vi "Multiply.vi"(2 "SampleFreq":dbl, 7 "Array in":cdb[](array[numeric]), 13 "MultiplyFreq":dbl) -> (8 "Array out":cdb[](array[numeric]))   [LabVIEW 2020]
uses:
  <vilib>/Analysis/NI_AAL_Angle.lvlib
  <vilib>/Analysis/coordinate.llb/Wrap Angle (scalar).vi
  <vilib>/Analysis/NI_AALPro.lvlib
  <vilib>/Analysis/2dsp.llb/Inverse Complex FFT.vi
  <vilib>/Analysis/2dsp.llb/Complex FFT.vi
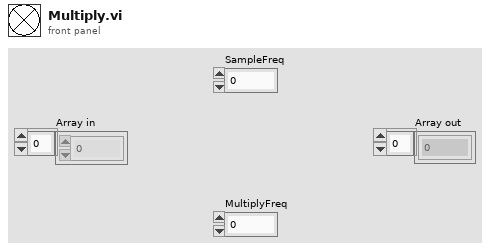
[diagram p1: front panel]
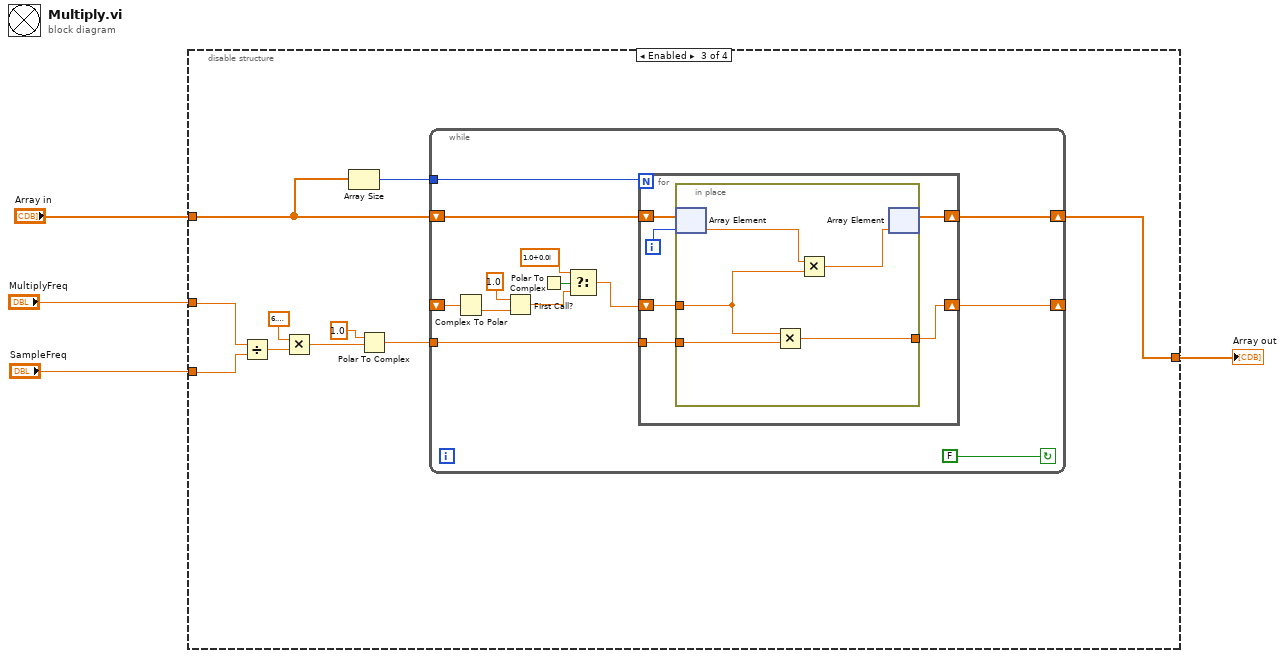
[diagram p0: block diagram]
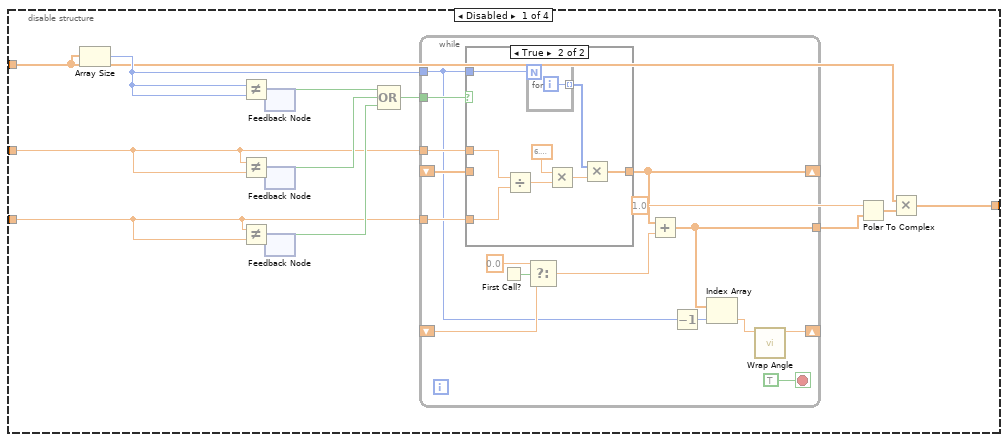
[diagram p2: hidden frame]
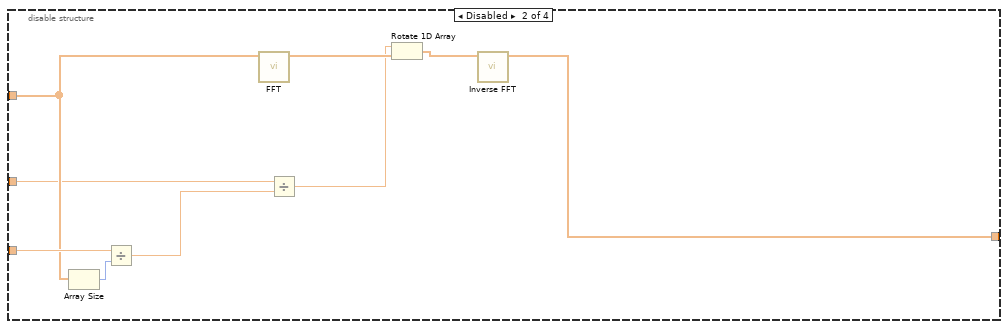
[diagram p4: hidden frame]
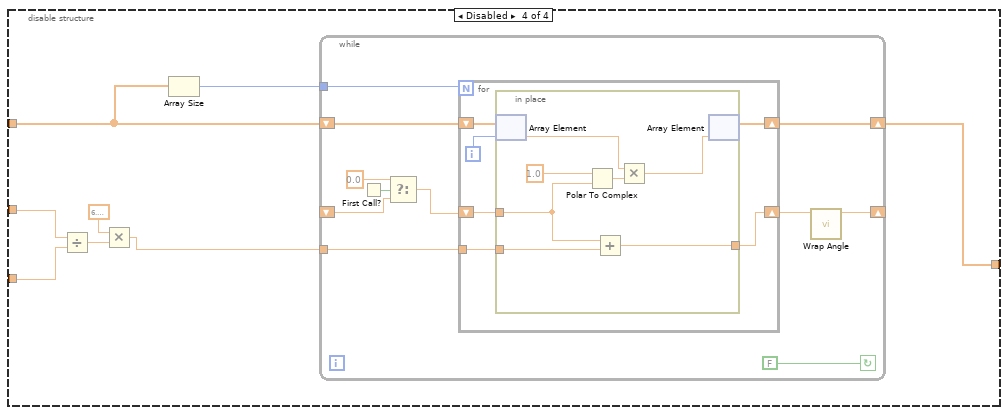
[diagram p5: hidden frame]
diagram:
  n1 = disable-structure shown="Enabled" {
    disable-tunnel: "MultiplyFreq" -> [w11 w50 w57 w89]
    disable-tunnel: "SampleFreq" -> [w10 w53 w58 w90]
    disable-tunnel: "Array in" -> [w6 w51 w62 w94]
    disable-tunnel: [w5 w45 w61 w93] -> w2
    frame Disabled {
      n2 = Array Size(array=w6) -> (size(s)=w12:i32)
      n3 = feedback #1() -> (w17:i32)  [unwired: 1 in]
      n4 = Not Equal?(x=w12, y=w17) -> (x != y?=w15:bool)
      n5 = feedback-in #1(w12) -> ()
      n6 = feedback #2() -> (w18:dbl)  [unwired: 1 in]
      n7 = Not Equal?(x=w11, y=w18) -> (x != y?=w14:bool)
      n8 = feedback-in #2(w11) -> ()
      n9 = feedback #3() -> (w19:dbl)  [unwired: 1 in]
      n10 = Not Equal?(x=w10, y=w19) -> (x != y?=w16:bool)
      n11 = feedback-in #3(w10) -> ()
      n12 = Compound Arithmetic op=OR(w15, w14, w16) -> (w13:bool)
      n13 = while {
        tunnel: w13 -> [w31]
        tunnel: w12 -> [w21]
        tunnel: w11 -> [w32]
        tunnel: w10 -> [w33]
        shift-right: [w26] -> _
        shift-left: _ -> [w30]
        shift-right: [w25] -> _
        shift-left: _ -> [w27]
        tunnel: [w20] -> w9
        stop <- TRUE stop-if-true
        n14 = case shown="True" w31 {
          tunnel: w21 -> [_ w43]
          tunnel: w33 -> [_ w40]
          tunnel: w32 -> [_ w39]
          tunnel: [w35 w36] -> w26
          tunnel: w30 -> [w35 _]
          frame False {
          }
          frame True {
            n15 = Divide(x=w39, y=w40) -> (x/y=w42:dbl)
            n16 = for {
              N: w43 -> [_]
              tunnel: [w44] -> w37 mode=indexing
              i -> [w44]
            }
            n17 = Multiply(x=6.283185307179586, y=w42) -> (x*y=w38:dbl)
            n18 = Multiply(x=w37, y=w38) -> (x*y=w36:dbl[])
          }
        }
        n19 = First Call?() -> (First Call?: T/F=w29:bool)
        n20 = Select(t=0.0, s=w29, f=w27) -> (s? t:f=w24:dbl)
        n21 = Add(x=w26, y=w24) -> (x+y=w20:dbl[])
        n22 = Decrement(x=w21) -> (x-1=w22:i32)
        n23 = Index Array(array=w20, index=w22) -> (element=w23:dbl)
        n24 = call-poly <vilib>:"Wrap Angle.vi"("angle in"=w23) -> ("angle out"=w25:dbl)  [unwired: 9 in, 1 out]
      }
      n25 = Polar To Complex(1:w9, 2:1.0 ("r")) -> (0:w7:cdb[])
      n26 = Multiply(x=w6, y=w7) -> (x*y=w5:cdb[])
    }
    frame Disabled {
      n27 = Array Size(array=w51) -> (size(s)=w52:i32)
      n28 = Divide(x=w53, y=w52) -> (x/y=w49:dbl)
      n29 = call-poly <vilib>:"FFT.vi"("X"=w51) -> ("FFT {X}"=w48:cdb[])  [unwired: 9 in, 1 out]
      n30 = Divide(x=w50, y=w49) -> (x/y=w46:dbl)
      n31 = Rotate 1D Array(1:w48, 2:w46) -> (0:w47:cdb[])
      n32 = call-poly <vilib>:"Inverse FFT.vi"("FFT {X}"=w47) -> ("X"=w45:cdb[])  [unwired: 9 in, 1 out]
    }
    frame Enabled {
      n33 = Divide(x=w57, y=w58) -> (x/y=w60:dbl)
      n34 = Multiply(x=6.283185307179586, y=w60) -> (x*y=w55:dbl)
      n35 = Array Size(array=w62) -> (size(s)=w63:i32)
      n36 = Polar To Complex(1:w55, 2:1.0 ("r")) -> (0:w54:cdb)
      n37 = while {
        tunnel: w63 -> [w75]
        tunnel: w54 -> [w73]
        shift-right: [w76] -> w61
        shift-left: w62 -> [w74]
        shift-right: [w68] -> _
        shift-left: _ -> [w67]
        stop <- FALSE continue-if-true
        n38 = Complex To Polar(r * e^(i*theta)=w67) -> (theta=w66:dbl)  [unwired: 1 out]
        n39 = Polar To Complex(1:w66, 2:1.0 ("r")) -> (0:w64:cdb)
        n40 = First Call?() -> (First Call?: T/F=w72:bool)
        n41 = Select(t=cdb 1.0+0.0i, s=w72, f=w64) -> (s? t:f=w69:cdb)
        n42 = for {
          N: w75 -> [_]
          shift-right: [w77] -> w76
          shift-left: w74 -> [w82]
          tunnel: w73 -> [w80]
          shift-right: [w79] -> w68
          shift-left: w69 -> [w78]
          i -> [w81]
          n43 = in-place {
            in-place-border: w80 -> [w87]
            in-place-border: [w84] -> w79
            in-place-border: w78 -> [w83]
            n44 = in-place-array #4(w82, w81) -> (w86:cdb)
            n45 = Multiply(x=w83, y=w87) -> (x*y=w84:cdb)
            n46 = Multiply(x=w86, y=w83) -> (x*y=w85:cdb)
            n47 = in-place-array #4(w85) -> (w77:cdb[])  [unwired: 1 out]
          }
        }
      }
    }
    frame Disabled {
      n48 = Divide(x=w89, y=w90) -> (x/y=w92:dbl)
      n49 = Multiply(x=6.283185307179586, y=w92) -> (x*y=w88:dbl)
      n50 = Array Size(array=w94) -> (size(s)=w95:i32)
      n51 = while {
        tunnel: w95 -> [w105]
        tunnel: w88 -> [w103]
        shift-right: [w106] -> w93
        shift-left: w94 -> [w104]
        shift-right: [w96] -> _
        shift-left: _ -> [w101]
        stop <- FALSE continue-if-true
        n52 = First Call?() -> (First Call?: T/F=w102:bool)
        n53 = Select(t=0.0, s=w102, f=w101) -> (s? t:f=w98:dbl)
        n54 = for {
          N: w105 -> [_]
          shift-right: [w107] -> w106
          shift-left: w104 -> [w112]
          tunnel: w103 -> [w110]
          shift-right: [w109] -> w97
          shift-left: w98 -> [w108]
          i -> [w111]
          n55 = in-place {
            in-place-border: w110 -> [w119]
            in-place-border: [w113] -> w109
            in-place-border: w108 -> [w118]
            n56 = in-place-array #5(w112, w111) -> (w115:cdb)
            n57 = Polar To Complex(1:w118, 2:1.0 ("r")) -> (0:w116:cdb)
            n58 = Add(x=w118, y=w119) -> (x+y=w113:dbl)
            n59 = Multiply(x=w115, y=w116) -> (x*y=w114:cdb)
            n60 = in-place-array #5(w114) -> (w107:cdb[])  [unwired: 1 out]
          }
        }
        n61 = call-poly <vilib>:"Wrap Angle.vi"("angle in"=w97) -> ("angle out"=w96:dbl)  [unwired: 9 in, 1 out]
      }
    }
  }
  "Array out" <- w2
